vi "digitalwffromfile.vi"(1 "Matlab wave file":path, 2 "Sampling frequency (Hz)":dbl) -> (0 "digital waveform":digitalwaveform(waveform))   [LabVIEW 2015]
uses:
  <vilib>/Utility/file.llb/Read Delimited Spreadsheet (DBL).vi
  <vilib>/Waveform/DWDTOps.llb/DWDT Analog to Digital.vi
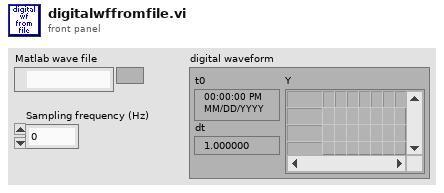
[diagram p1: front panel]
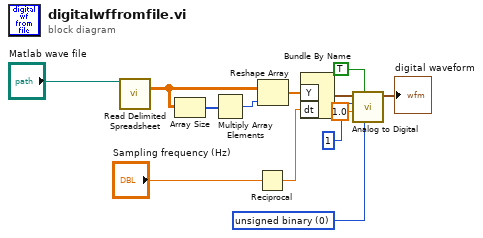
[diagram p0: block diagram]
diagram:
  w11 = u16 0 items=["unsigned binary", "offset binary", "2's complement"] ("data format (offset binary)")
  n1 = call-poly <vilib>:"Read Delimited Spreadsheet.vi"("file path (dialog if empty)"="Matlab wave file") -> ("all rows"=w7:dbl[][])  [unwired: 9 in, 5 out]
  n2 = Array Size(array=w7) -> (size(s)=w6:i32[])
  n3 = Multiply Array Elements(1:w6) -> (0:w5:i32)
  n4 = Reciprocal(x="Sampling frequency (Hz)") -> (1/x=w3:dbl)
  n5 = Reshape Array(w7, w5) -> (w4:dbl[])
  n6 = Bundle By Name("Y"=w4, "dt"=w3) -> (w13:waveform(dbl))  [unwired: 1 in]
  n7 = call-poly <vilib>:"Analog to Digital.vi"("data format (offset binary)"=w11, "compress digital (T)"=TRUE, "full-scale range (pk-pk)"=1.0, "resolution (16 bit)"=1, "analog waveform"=w13) -> ("digital waveform"=→"digital waveform":digitalwaveform)  [unwired: 3 in, 3 out]
